vi "SortRank&place.vi"() -> ()   [LabVIEW 2019]
panel:
  in  "字符串":string
  in  "布尔":bool
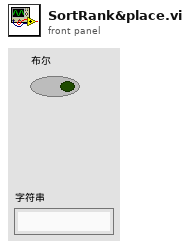
[diagram p1: front panel]
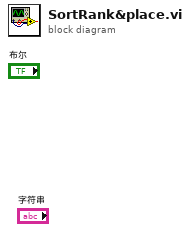
[diagram p0: block diagram]
diagram:
